vi "실습2-3수식노드.vi"() -> ()   [LabVIEW 2014]
panel:
  out "숫자형":dbl format="%#_20g"
  out "웨이브폼 그래프":dbl[](graph)
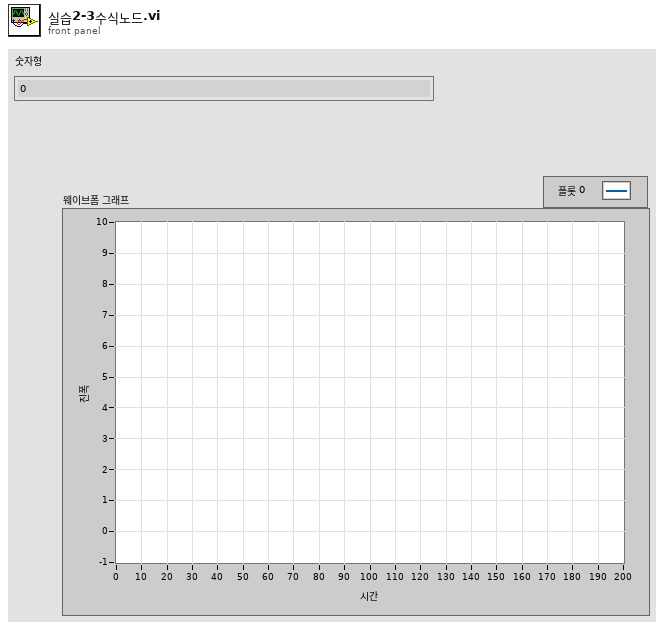
[diagram p1: front panel]
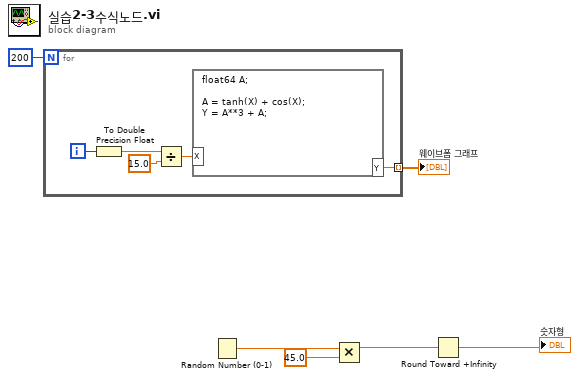
[diagram p0: block diagram]
diagram:
  n1 = for {
    N: 200 -> [_]
    tunnel: [w7] -> w5 mode=indexing
    i -> [w11]
    n2 = To Double Precision Float(number=w11) -> (double precision float=w10:dbl)
    n3 = Divide(x=w10, y=15.0) -> (x/y=w8:dbl)
    n4 = formula code="float64 A;\n\nA = tanh(X) + cos(X);\nY = A**3 + A;"("X"=w8) -> ("Y"=w7:dbl)
  }
  "웨이브폼 그래프" <- w5
  n5 = Random Number (0-1)() -> (number: 0 to 1=w4:dbl)
  n6 = Multiply(x=w4, y=45.0) -> (x*y=w3:dbl)
  n7 = Round Toward +Infinity(x=w3) -> (ceil(x): smallest int >= x=→"숫자형":dbl)
